vi "Initialize.vi"(0 "resources":string, 1 "https?":bool, 2 "slsc type":T1, 5 "Hostname/IP":string, 7 "Port":u16, 11 "error in (no error)":errorcluster, 12 "username":string, 13 "password":string) -> (4 "SLSC Remote out":refnum<class "SLSC Remote.lvclass">, 15 "error out":errorcluster)   [LabVIEW 2015, in "SLSC Remote.lvclass"]
uses:
  SLSC Remote.lvclass
  SLSC Interface Class/slsc type.ctl
  <vilib>/httpClient/POSTBuffer.vi
  <vilib>/NI/i3 JSON/JSON Parsing/Get Object Parameter Files/Get Object Parameter - String.vi
  <vilib>/httpClient/LabVIEWHTTPClient.lvlib
  <vilib>/NI/i3 JSON/i3-json.lvlib
  <vilib>/NI/NI JSONRPC Server Framework/Classes/Server/JSONRPC Server.lvclass
  SLSC Interface Class/SLSC Interface.lvclass
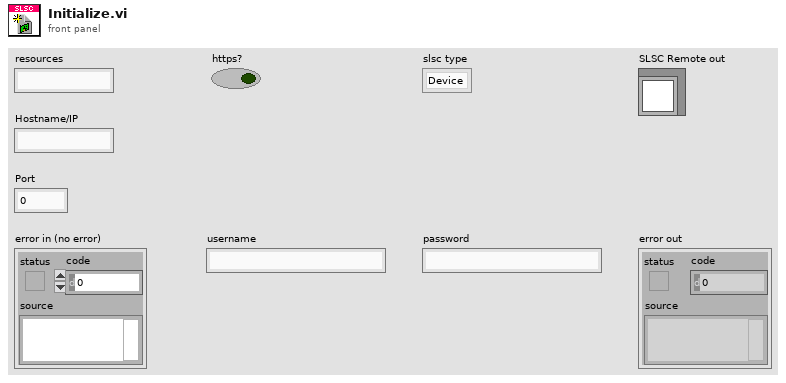
[diagram p1: front panel]
types:
  T1 = typedef "SLSC Interface.lvclass/slsc type.ctl" = enum16{"Device", "NVMEM Area", "Physical Channel", "None"}
  T2 = typedef "LabVIEWHTTPClient.lvlib/ClientHandle.ctl" = refnum<k1>
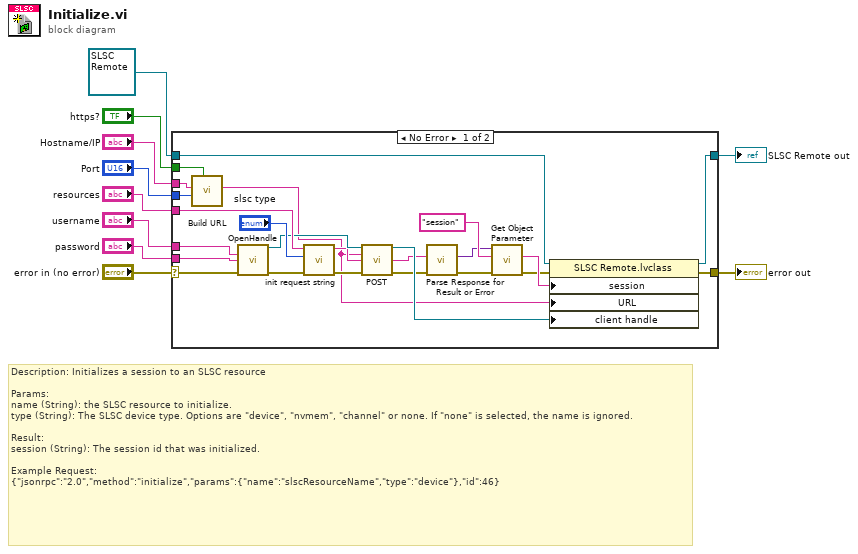
[diagram p0: block diagram]
diagram:
  # "Description: Initializes a session to an SLSC resource\n\nParams:\nname (String): the SLSC resource to initialize.\ntype (String): The SLSC device type. Options are \"device\", \"nvmem\", \"channel\" or none. If \"none\" is selected, the name is ignored.\n\nResult:\nsession (String): The session id that was initialized.\n\nExample Request: \n{\"jsonrpc\":\"2.0\",\"method\":\"initialize\",\"params\":{\"name\":\"slscResourceName\",\"type\":\"device\"},\"id\":46}"
  n1 = case shown="No Error" "error in (no error)" {
    selector: "error in (no error)" -> [w29 w36]
    tunnel: [w32 w36] -> w10
    tunnel: [w33 w35] -> w8
    tunnel: refnum<class "SLSC Remote.lvclass"> refnum ("SLSC Local in") -> [w34 w35]
    tunnel: "resources" -> [w27 _]
    tunnel: "username" -> [w31 _]
    tunnel: "password" -> [w30 _]
    tunnel: "https?" -> [w20 _]
    tunnel: "Hostname/IP" -> [w19 _]
    tunnel: "Port" -> [w18 _]
    frame No Error {
      n2 = call "Build URL.vi"("https?"=w20, "Port"=w18, "Hostname/IP"=w19) -> ("URL"=w16:string)  [unwired: 8 in]
      n3 = call <vilib>:"OpenHandle.vi"("username"=w31, "password"=w30, "error in (no error)"=w29) -> ("client handle out"=w25:T2, "error out"=w24:errorcluster)  [unwired: 11 in]
      n4 = call "init request string.vi"("error in (no error)"=w24, "slsc type"="slsc type", "resource"=w27) -> ("error out"=w26:errorcluster, "Request String"=w17:string)  [unwired: 7 in]
      n5 = call-poly <vilib>:"POST.vi"("client handle"=w25, "url"=w16, "buffer"=w17, "error in (no error)"=w26) -> ("client handle out"=w23:T2, "body"=w15:string, "error out"=w11:errorcluster)  [unwired: 8 in, 1 out]
      n6 = call <vilib>:"Parse Response for Result or Error.vi"("error in"=w11, "Response String In"=w15) -> ("error out"=w12:errorcluster, "Result or Error Data"=w13:variant)  [unwired: 7 in, 1 out]
      n7 = call-poly <vilib>:"Get Object Parameter.vi"("error in (no error)"=w12, "Parameter Name"="session", "JSON Tree In (JSON Object)"=w13) -> ("error out"=w21:errorcluster, "String Value"=w22:string)  [unwired: 5 in, 2 out]
      n8 = property class="SLSC Remote.lvclass"(reference=w34, error in=w21, "session"=w22, "URL"=w16, "client handle"=w23) -> (reference out=w33:refnum<class "SLSC Remote.lvclass">, error out=w32:errorcluster)
    }
    frame Error {
    }
  }
  "error out" <- w10
  "SLSC Remote out" <- w8
